vi "Agilent_Abort.vi"(8 "error in (no error)":errorcluster, 11 "VISA resource name":refnum<visa-resource-name>) -> (0 "error out":errorcluster, 3 "VISA resource name out":refnum<visa-resource-name>)   [LabVIEW 2020]
doc: "This VI configures the number of waveforms that the oscilloscope acquires and averages. After the oscilloscope acquires as many waveforms as you specify, it returns to the idle state. \n\nNotes:\n(1) Set the acquisition type to 2: Average before you call this VI. To set the acquisition type, call the ag6000 Configure Acquisition Type.vi."
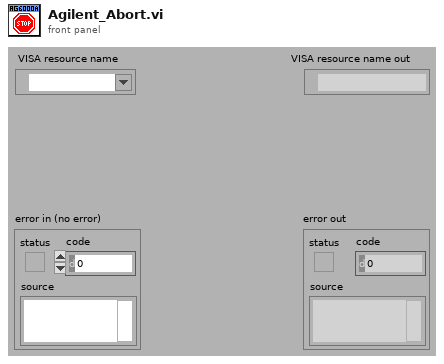
[diagram p1: front panel]
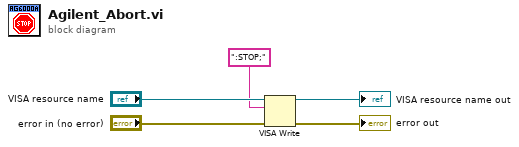
[diagram p0: block diagram]
diagram:
  n1 = VISA Write(VISA resource name="VISA resource name", write buffer=":STOP;", error in (no error)="error in (no error)") -> (VISA resource name out=→"VISA resource name out":refnum<visa-resource-name>, error out=→"error out":errorcluster)  [unwired: 1 out]
